vi "SimpleMotorFF_MinAchieveAccel.vi"(9 "Velocity":dbl, 10 "MaxVoltage":dbl, 11 "SIMPLE_MOTOR_FF":T1 {"Ka" format="%13.4f"; "Kv" format="%13.4f"; "Ks" format="%13.4f"}) -> (3 "MinAccel":dbl)   [LabVIEW 2019, in "Trajectory_Library.lvlib"]
doc: "Calculates the minimum achievable acceleration given a maximum voltage supply and a velocity. Useful for ensuring that velocity and acceleration constraints for a trapezoidal profile are simultaneously achievable - enter the velocity constraint, and this will give you a simultaneously-achievable acceleration constraint.\n\nParameters:\n - Simple_Motor_FF - Data structure containing constants\n - maxVoltage -The maximum voltage that can be supplied to the motor.\n - velocity - The velocity of the motor.\n\nReturns:\n - MinAccel - The minimum possible acceleration at the given velocity."
uses:
  Trajectory_Library.lvlib
  SIMPLE_MOTOR_FF.ctl
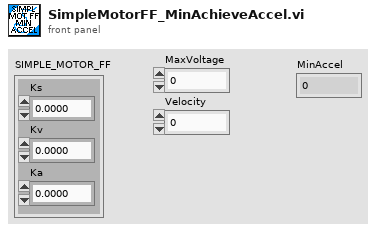
[diagram p1: front panel]
types:
  T1 = typedef "Trajectory_Library.lvlib/SIMPLE_MOTOR_FF.ctl" = cluster{"Ks":dbl, "Kv":dbl, "Ka":dbl}
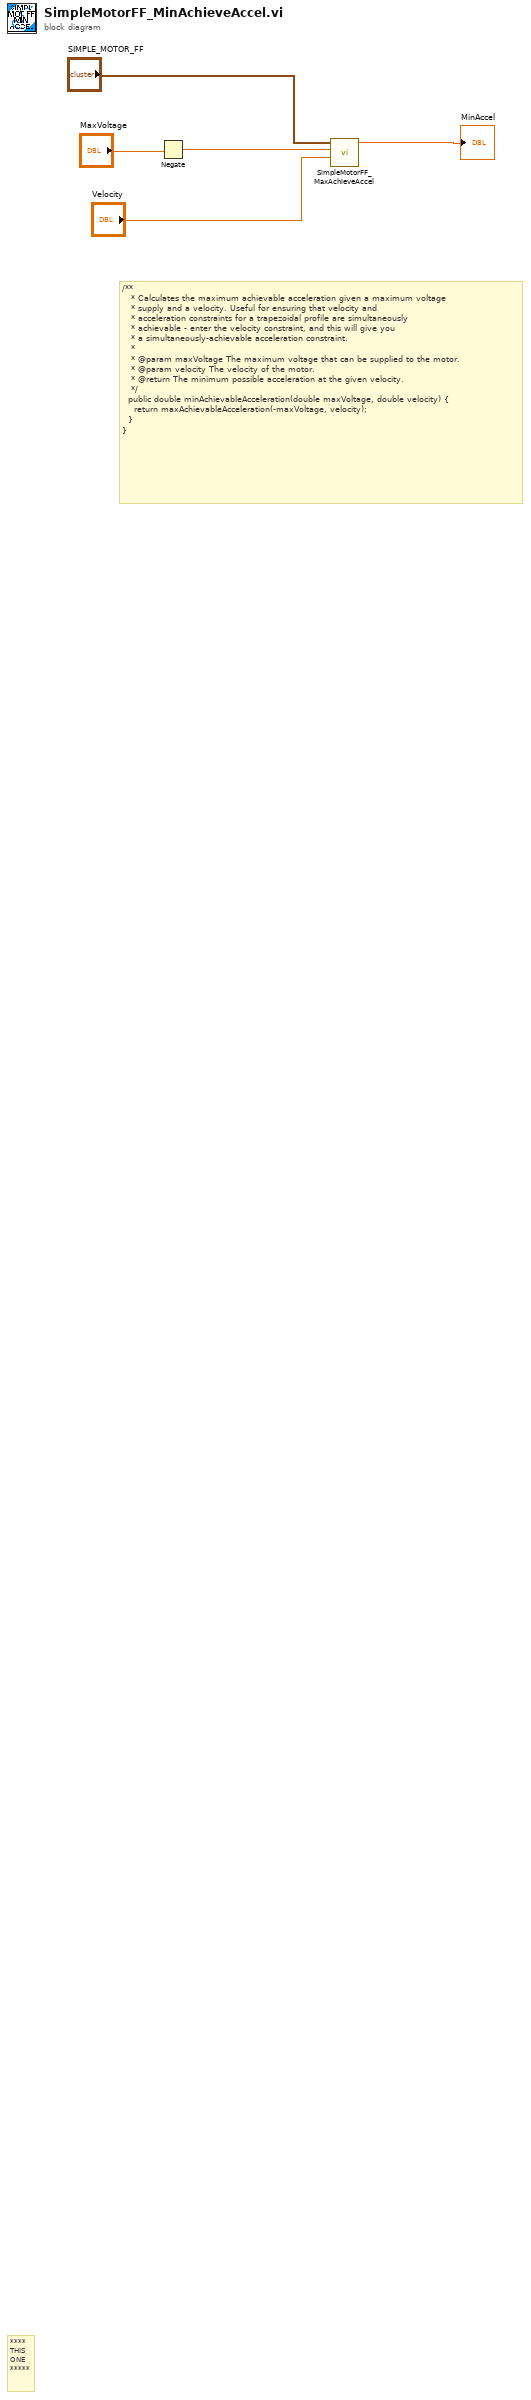
[diagram p0: block diagram]
diagram:
  # "/**\n   * Calculates the maximum achievable acceleration given a maximum voltage\n   * supply and a velocity. Useful for ensuring that velocity and\n   * acceleration constraints for a trapezoidal profile are simultaneously\n   * achievable - enter the velocity constraint, and this will give you\n   * a simultaneously-achievable acceleration constraint.\n   *\n   * @param maxVoltage The maximum voltage that can be supplied to the motor.\n   * @param velocity The velocity of the motor.\n   * @return The minimum possible acceleration at the given velocity.\n   */\n  public double minAchievableAcceleration(double maxVoltage, double velocity) {\n    return maxAchievableAcceleration(-maxVoltage, velocity);\n  }\n}"
  # "****\nTHIS\nONE\n*****"
  n1 = Negate(x="MaxVoltage") -> (-x=w3:dbl)
  n2 = call "SimpleMotorFF_MaxAchieveAccel.vi"("Velocity"="Velocity", "MaxVoltage"=w3, "SIMPLE_MOTOR_FF"="SIMPLE_MOTOR_FF") -> ("MaxAccel"=→"MinAccel":dbl)  [unwired: 8 in]
